vi "Pcre2PatternInfoCaptureCount8.vi"(8 "error in":errorcluster, 11 "pCode":u64 format="%.0x") -> (0 "error out":errorcluster, 2 "CaptureCount":u32, 3 "pCode":u64 format="%.0x")   [LabVIEW 2021, in "libpcre2-8.lvlib"]
uses:
  libpcre2-8.lvlib
  Pcre2FnkCallError.vi
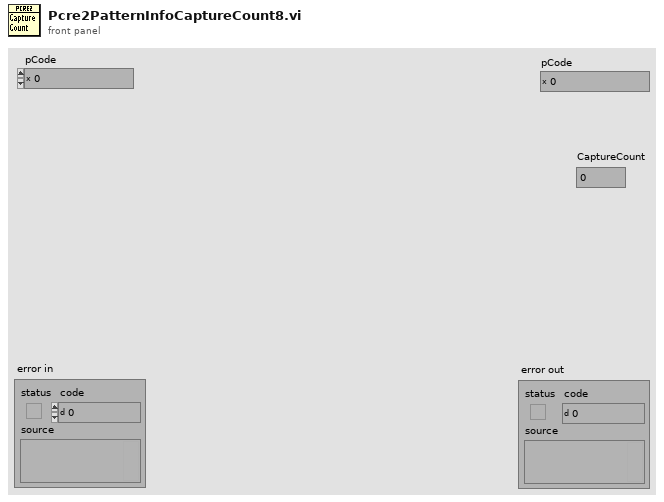
[diagram p1: front panel]
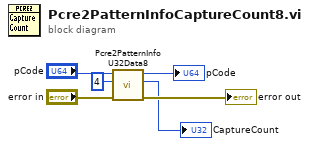
[diagram p0: block diagram]
diagram:
  n1 = call "Pcre2PatternInfoU32Data8.vi"("error in"="error in", "What"=u32 4, "pCode"="pCode") -> ("error out"=→"error out":errorcluster, "Info"=→"CaptureCount":u32, "pCode"=→"pCode":u64)  [unwired: 6 in]
